vi "Add Rows (String).vi"(8 "error in (no error)":errorcluster, 9 "String Data":string[][](array[string]), 11 "DataTable in":refnum<class "DataTable.lvclass">) -> (0 "error out":errorcluster, 3 "DataTable out":refnum<class "DataTable.lvclass">)   [LabVIEW 2013, in "DataGrid.lvlib" / "DataTable.lvclass"]
doc: "This allows any number of rows to be added to the datatable. The data must match the columns defined for the grid."
uses:
  DataTable.lvclass
  DataTable.lvclass/DataTable.ctl
  System.Data
  GridColumn/GridColumn.lvclass/GridColumn.ctl
  GridColumn/Read datatype.vi
  GridColumn/Read Params.vi
  GridColumn/Read Name.vi
  GridColumn/GridColumn.lvclass
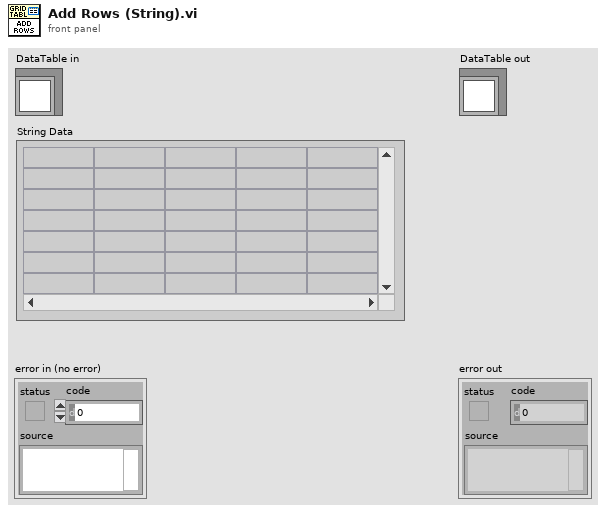
[diagram p1: front panel]
types:
  T1 = typedef "DataGrid.lvlib/GridColumn.lvclass/ColumnType.ctl" = enum16{"string", "image", "check", "numeric", "timestamp", "button", "combo", "link"}
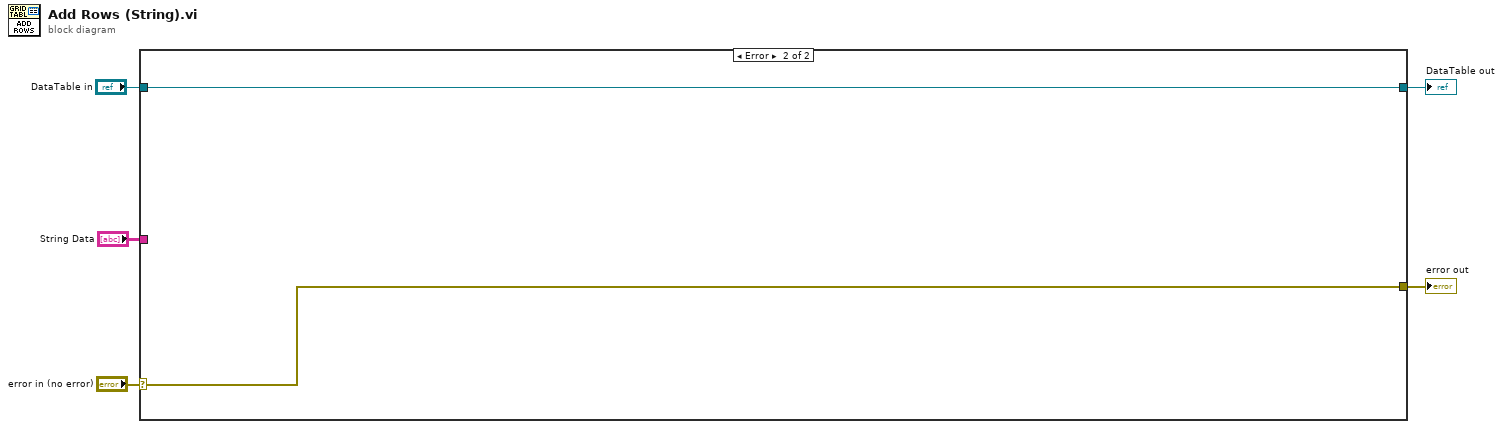
[diagram p0: block diagram]
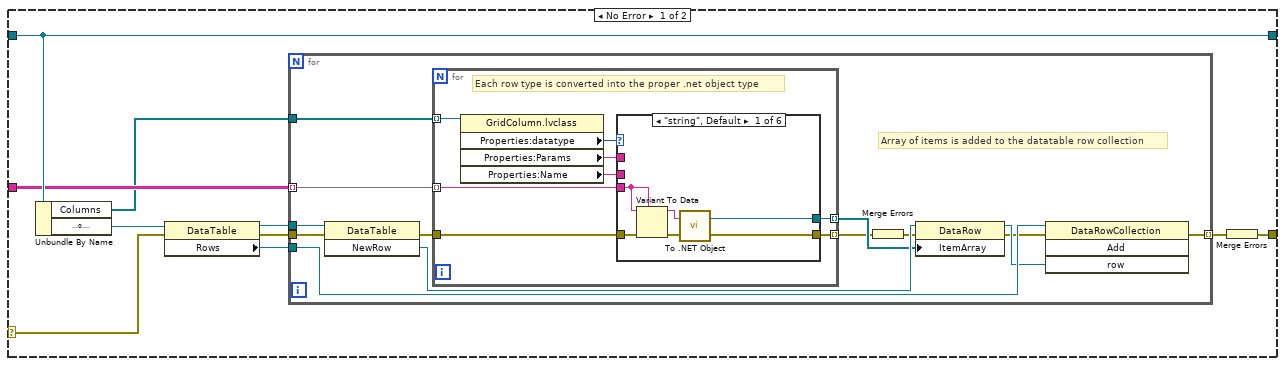
[diagram p2: hidden frame]
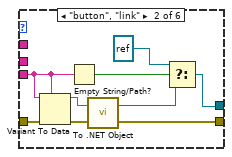
[diagram p3: hidden frame]
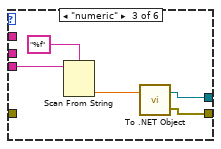
[diagram p4: hidden frame]
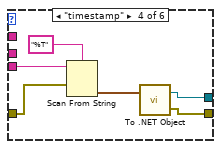
[diagram p5: hidden frame]
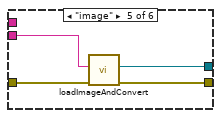
[diagram p6: hidden frame]
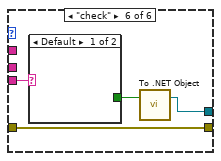
[diagram p7: hidden frame]
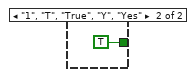
[diagram p8: hidden frame]
diagram:
  n1 = case shown="Error" "error in (no error)" {
    selector: "error in (no error)" -> [w11 w72]
    tunnel: [w12 w73] -> w3
    tunnel: "DataTable in" -> [w12 w73]
    tunnel: "String Data" -> [w10 _]
    tunnel: [w7 w72] -> w1
    frame No Error {
      n2 = Unbundle By Name(w12) -> ("Columns"=w6:refnum<class "GridColumn.lvclass">[], "DataTable"=w9:refnum<k24>)
      n3 = property class="DataTable"(reference=w9, error in=w11) -> (reference out=w8:refnum<k24>, error out=w15:errorcluster, "Rows"=w14:refnum<k24>)
      n4 = for {
        tunnel: w14 -> [w27]
        tunnel: w8 -> [w28]
        tunnel: [w26] -> w13 mode=indexing
        tunnel: w10 -> [w25] mode=indexing
        tunnel: w15 -> [w17]
        tunnel: w6 -> [w16]
        # "Array of items is added to the datatable row collection"
        n5 = invoke class="DataTable" method="NewRow"(reference=w28, error in=w17) -> (error out=w24:errorcluster, "NewRow"=w23:refnum<k24>)  [unwired: 1 in, 1 out]
        n6 = for {
          tunnel: w25 -> [w36] mode=indexing
          tunnel: [w35] -> w21 mode=indexing
          tunnel: w24 -> [w34]
          tunnel: [w33] -> w20 mode=indexing
          tunnel: w16 -> [w32] mode=indexing
          # "Each row type is converted into the proper .net object type"
          n7 = property class="GridColumn.lvclass"(reference=w32) -> ("Properties:datatype"=w31:T1, "Properties:Params"=w30:string, "Properties:Name"=w29:string)  [unwired: 1 in, 2 out]
          n8 = case shown="\"string\", Default" w31 {
            tunnel: w36 -> [w38 w47 w54 w60 w66 w68]
            tunnel: [w37 w44 w55 w61 w65 w69] -> w35
            tunnel: w34 -> [w41 w50 _ w58 w64 w70]
            tunnel: [w39 w48 w56 w62 w63 w70] -> w33
            tunnel: w30 -> [_ _ _ _ _ _]
            tunnel: w29 -> [_ _ _ _ _ _]
            frame "string", Default {
              n9 = Variant To Data(error in=w41, type=w38, Variant=w38) -> (data=w42:string, error out=w40:errorcluster)
              n10 = call <vilib>:"To .NET Object.vi"("error in (no error)"=w40, "anything"=w42) -> ("error out"=w39:errorcluster, ".NET object"=w37:refnum<k24>)
            }
            frame "button", "link" {
              n11 = Variant To Data(error in=w50, type=w47, Variant=w47) -> (data=w51:string, error out=w49:errorcluster)
              n12 = Empty String/Path?(string/path=w47) -> (empty?=w46:bool)
              n13 = call <vilib>:"To .NET Object.vi"("error in (no error)"=w49, "anything"=w51) -> ("error out"=w48:errorcluster, ".NET object"=w45:refnum<k24>)
              n14 = Select(t=refnum<k24> refnum, s=w46, f=w45) -> (s? t:f=w44:refnum<k24>)
            }
            frame "numeric" {
              n15 = Scan From String(format string="%f", input string=w54) -> (output 1=w52:dbl)  [unwired: 3 in, 3 out]
              n16 = call <vilib>:"To .NET Object.vi"("anything"=w52) -> ("error out"=w56:errorcluster, ".NET object"=w55:refnum<k24>)  [unwired: 1 in]
            }
            frame "timestamp" {
              n17 = Scan From String(format string="%T", input string=w60, error in=w58) -> (output 1=w57:timestamp)  [unwired: 2 in, 3 out]
              n18 = call <vilib>:"To .NET Object.vi"("anything"=w57) -> ("error out"=w62:errorcluster, ".NET object"=w61:refnum<k24>)  [unwired: 1 in]
            }
            frame "image" {
              n19 = call "loadImageAndConvert.vi"("error in (no error)"=w64, "name or relative path"=w66) -> ("error out"=w63:errorcluster, ".NET object"=w65:refnum<k24>)  [unwired: 8 in]
            }
            frame "check" {
              n20 = case shown="Default" w68 {
                tunnel: [_ TRUE] -> w67
                frame Default {
                }
                frame "1", "T", "True", "Y", "Yes" {
                }
              }
              n21 = call <vilib>:"To .NET Object.vi"("anything"=w67) -> (".NET object"=w69:refnum<k24>)  [unwired: 1 in, 1 out]
            }
          }
        }
        n22 = Merge Errors(w20) -> (w19:errorcluster)
        n23 = property class="DataRow"(reference=w23, error in=w19, "ItemArray"=w21) -> (reference out=w22:refnum<k24>, error out=w18:errorcluster)
        n24 = invoke class="DataRowCollection" method="Add"(reference=w27, error in=w18, "row"=w22) -> (error out=w26:errorcluster)  [unwired: 1 in, 3 out]
      }
      n25 = Merge Errors(w13) -> (w7:errorcluster)
    }
    frame Error {
    }
  }
  "error out" <- w1
  "DataTable out" <- w3
